vi "Read Cal Tone Port.vi"(8 "error in (no error)":errorcluster, 11 "SA Path in":refnum<class "SA Abstract Path.lvclass">) -> (0 "error out":errorcluster, 2 "Cal Tone Port":string, 3 "SA Path out":refnum<class "SA Abstract Path.lvclass">)   [LabVIEW 2023, in "RFFixtureCharact.Public.lvlib" / "SA Abstract Path.lvclass"]
uses:
  SA Abstract Path.lvclass
  SA Abstract Path.lvclass/SA Abstract Path.ctl
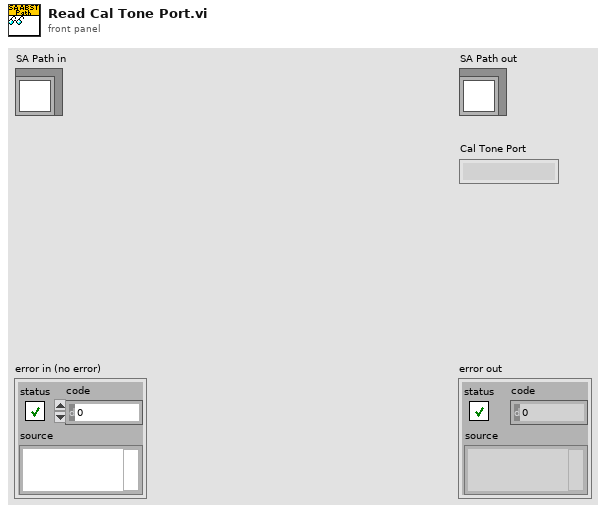
[diagram p1: front panel]
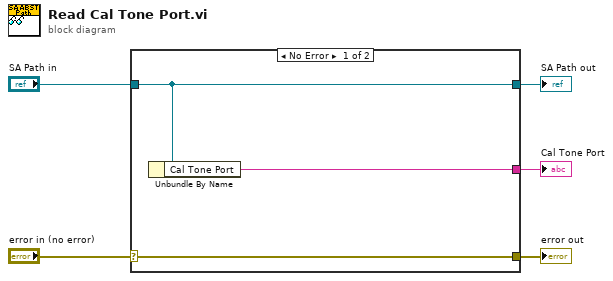
[diagram p0: block diagram]
diagram:
  n1 = case shown="No Error" "error in (no error)" {
    selector: "error in (no error)" -> [w8 w9]
    tunnel: [w8 w9] -> w4
    tunnel: [w7 w10] -> w2
    tunnel: "SA Path in" -> [w7 w10]
    tunnel: [w6 _] -> w1
    frame No Error {
      n2 = Unbundle By Name(w7) -> ("Cal Tone Port"=w6:string)
    }
    frame Error {
    }
  }
  "error out" <- w4
  "SA Path out" <- w2
  "Cal Tone Port" <- w1
